vi "Options Changed GFV .vi"(2 "Changed":bool, 3 "Previous Change No":i32, 6 "Action(Changed?)":T1(ring)=enum."Changed?", 7 "Setting ID":T2=enum."P 2") -> (16 "Settings Updated":bool, 17 "Change No":i32)   [LabVIEW 2011]
uses:
  Options PageID.ctl
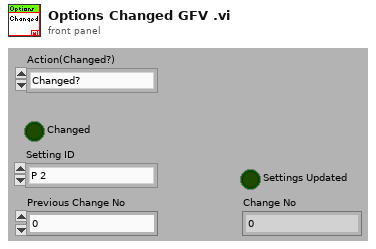
[diagram p1: front panel]
types:
  T1 = enum16{"Set Changed", "Changed?", "Init(numb in Prev..)"}
  T2 = typedef "Options PageID.ctl" = enum16{"P 1 (App)", "P 2", "P 3", "P 4", "P 5", "P 6 (Err)", "P 7 (Expert)", "P 8", "C 1", "C 2"}
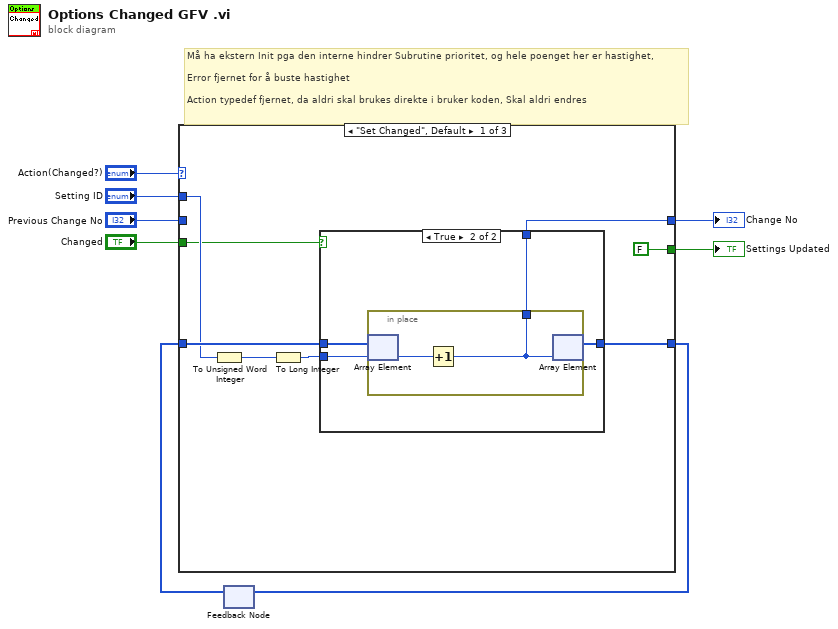
[diagram p0: block diagram]
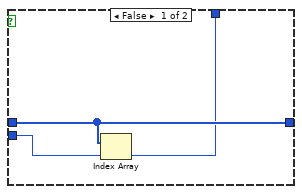
[diagram p2: hidden frame]
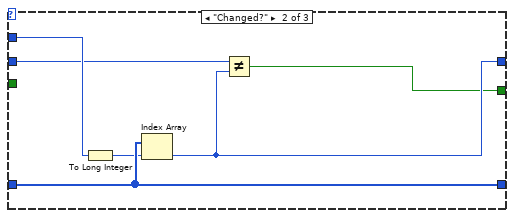
[diagram p3: hidden frame]
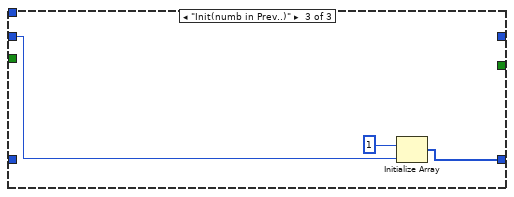
[diagram p4: hidden frame]
diagram:
  # "Må ha ekstern Init pga den interne hindrer Subrutine prioritet, og hele poenget her er hastighet,\n\nError fjernet for å buste hastighet\n\nAction typedef fjernet, da aldri skal brukes direkte i bruker koden, Skal aldri endres"
  n1 = feedback #1() -> (w1:i32[])  [unwired: 1 in]
  n2 = case shown="\"Set Changed\", Default" "Action(Changed?)" {
    tunnel: w1 -> [w16 w31 _]
    tunnel: [w15 w31 w32] -> w7
    tunnel: "Setting ID" -> [w14 w29 _]
    tunnel: "Previous Change No" -> [_ w27 w33]
    tunnel: [w11 w28 _] -> w4
    tunnel: [FALSE w26 _] -> w3
    tunnel: "Changed" -> [w10 _ _]
    frame "Set Changed", Default {
      n3 = To Unsigned Word Integer(number=w14) -> (unsigned 16bit integer=w9:u16)
      n4 = To Long Integer(number=w9) -> (32bit integer=w13:i32)
      n5 = case shown="True" w10 {
        tunnel: w16 -> [w18 w23]
        tunnel: [w18 w22] -> w15
        tunnel: w13 -> [w19 w21]
        tunnel: [w17 w20] -> w11
        frame False {
          n6 = Index Array(array=w18, index=w19) -> (element=w17:i32)
        }
        frame True {
          n7 = in-place {
            in-place-border: [w24] -> w20
            n8 = in-place-array #2(w23, w21) -> (w25:i32)
            n9 = Increment(x=w25) -> (x+1=w24:i32)
            n10 = in-place-array #2(w24) -> (w22:i32[])  [unwired: 1 out]
          }
        }
      }
    }
    frame "Changed?" {
      n11 = To Long Integer(number=w29) -> (32bit integer=w30:i32)
      n12 = Index Array(array=w31, index=w30) -> (element=w28:i32)
      n13 = Not Equal?(x=w27, y=w28) -> (x != y?=w26:bool)
    }
    frame "Init(numb in Prev..)" {
      n14 = Initialize Array(1, w33) -> (w32:i32[])
    }
  }
  "Change No" <- w4
  "Settings Updated" <- w3
  n15 = feedback-in #1(w7) -> ()
